vi "Command_verification_SA test.vi"(3 "time out":i32=40000, 4 "connection ID":refnum<k5>) -> (0 "Get_mea_condition":T1 {"RoiLateralSpan" format="%.2f"; "RoiLateralMin" format="%.2f"}, 1 "RLE data":string)   [LabVIEW 2016]
uses:
  TemperatureMeasure/Thermal_type.vi
panel:
  out "B-mode(Hout_Lout_Reg)":string[](array[string])
  in  "mea_condition_setting":T1 {"RoiLateralMin" format="%.2f"; "RoiLateralSpan" format="%.2f"}
  in  "error out":errorcluster
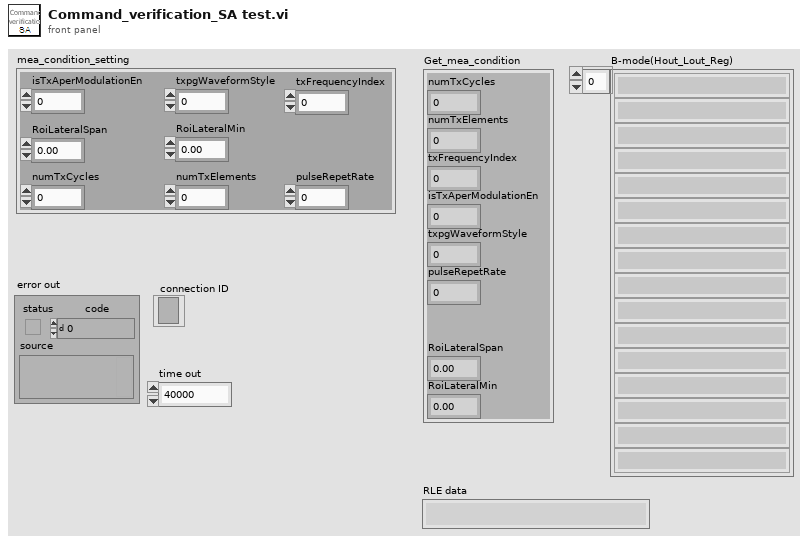
[diagram p1: front panel]
types:
  T1 = cluster{"numTxCycles":dbl, "numTxElements":i16, "txFrequencyIndex":i32, "isTxAperModulationEn":i16, "txpgWaveformStyle":i16, "pulseRepetRate":dbl, "RoiLateralSpan":dbl, "RoiLateralMin":dbl}
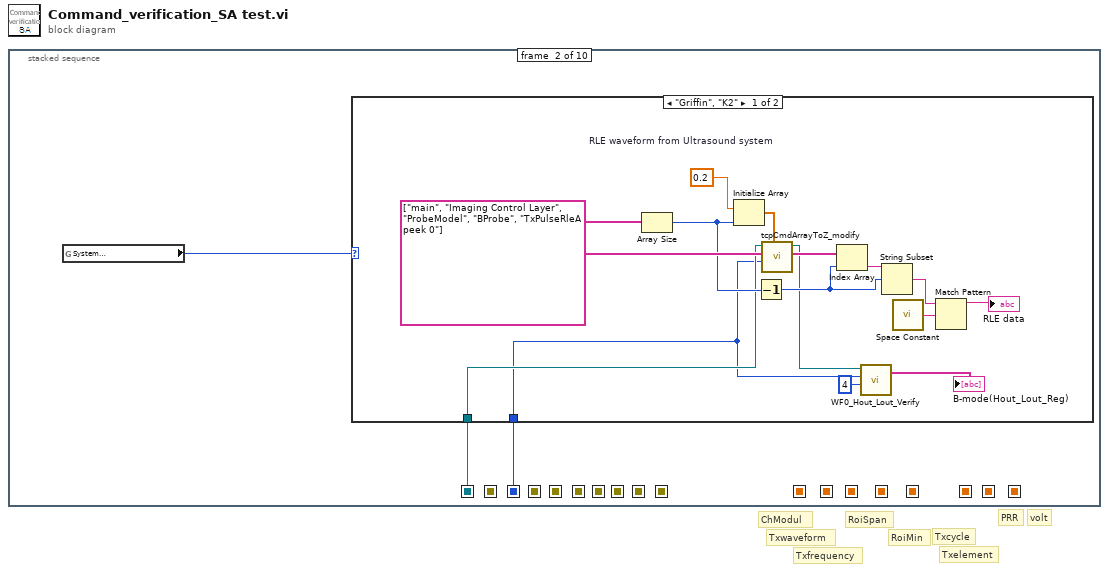
[diagram p0: block diagram]
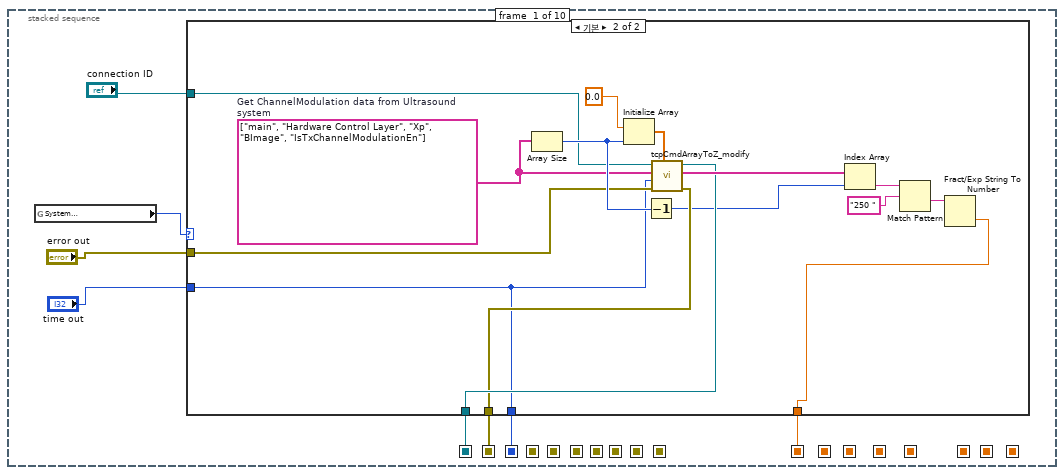
[diagram p2: hidden frame]
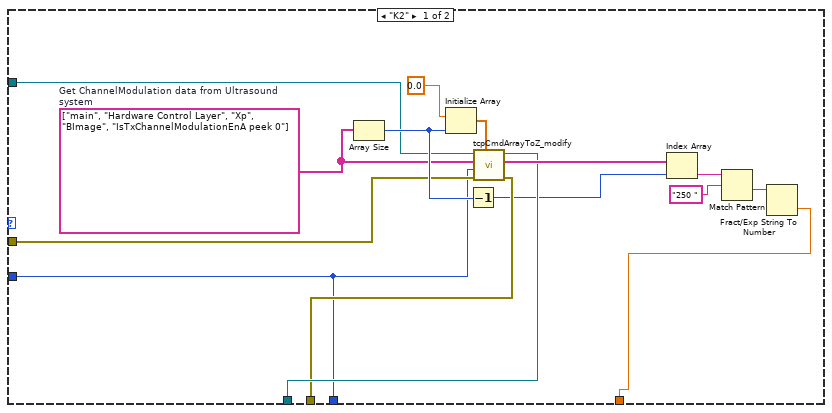
[diagram p3: hidden frame]
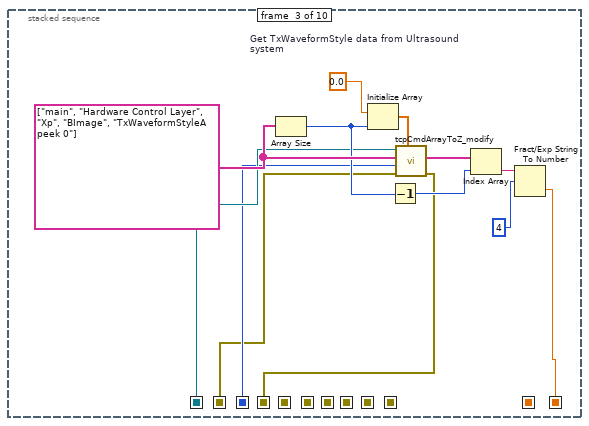
[diagram p5: hidden frame]
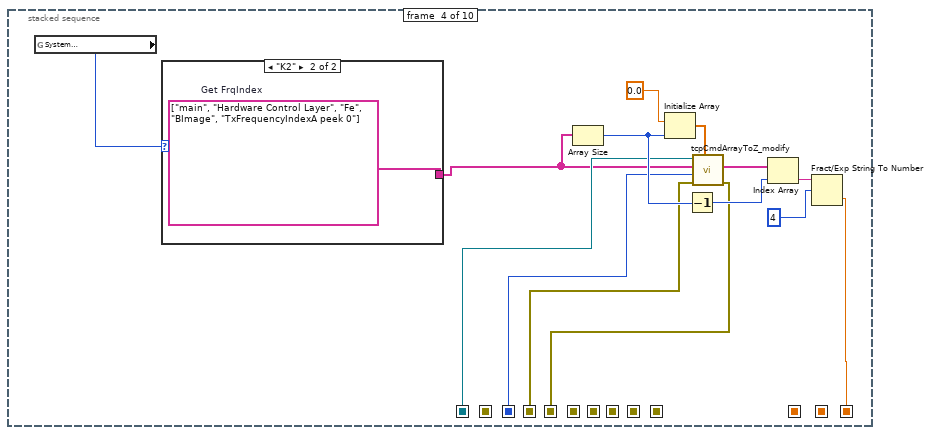
[diagram p6: hidden frame]
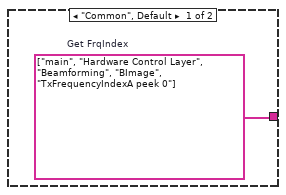
[diagram p7: hidden frame]
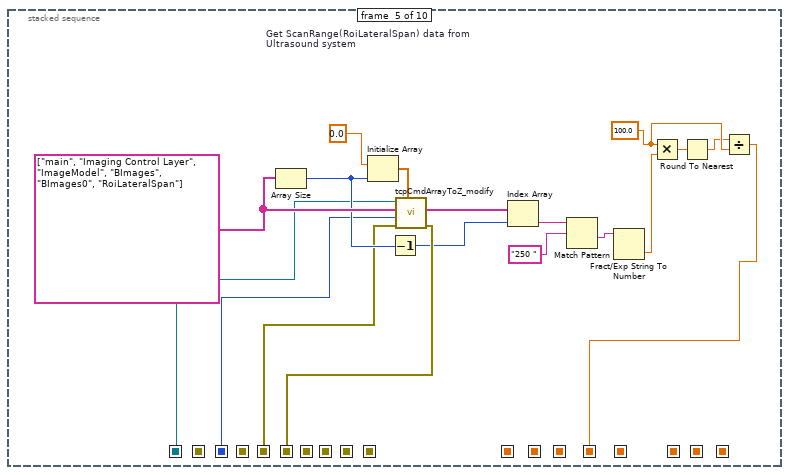
[diagram p8: hidden frame]
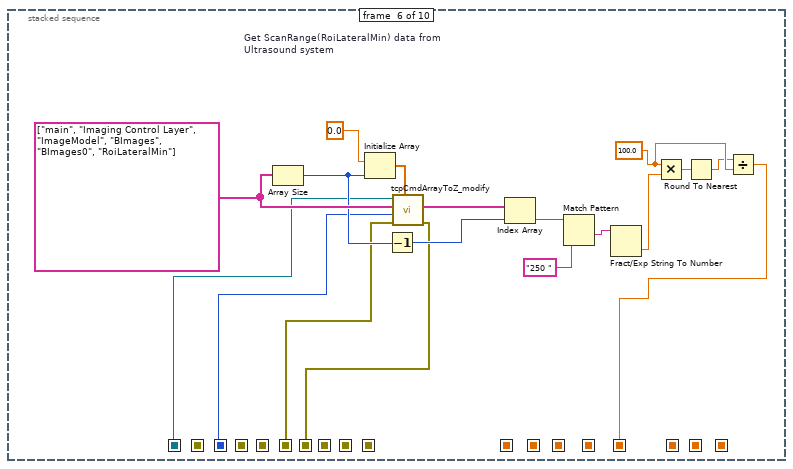
[diagram p9: hidden frame]
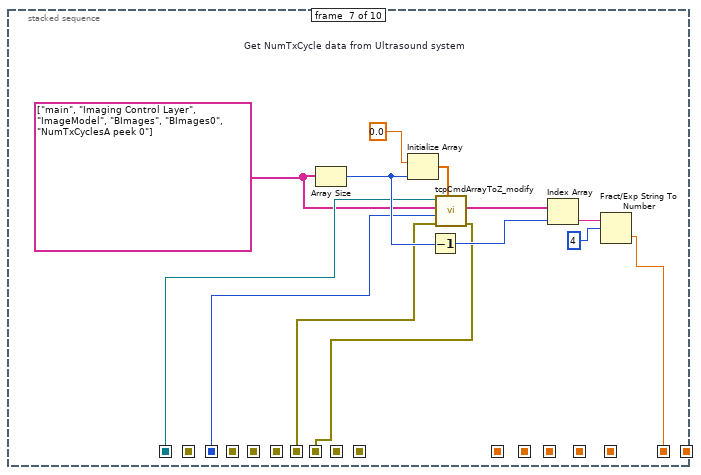
[diagram p10: hidden frame]
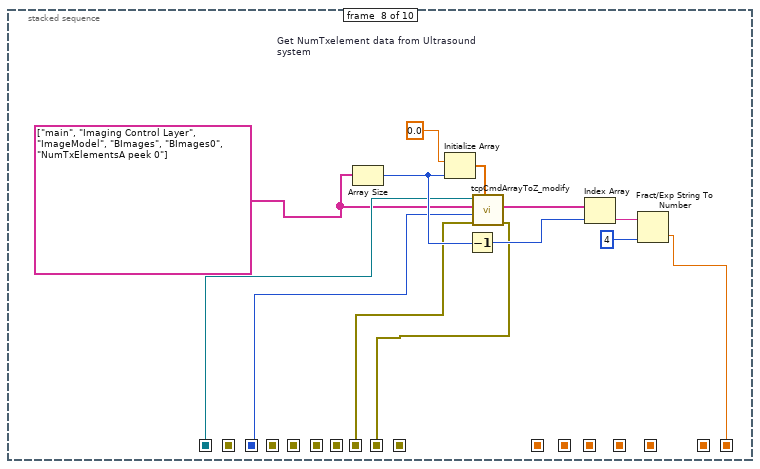
[diagram p11: hidden frame]
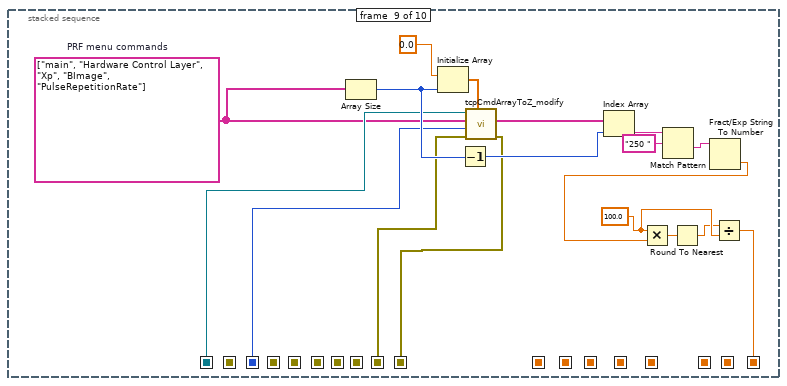
[diagram p12: hidden frame]
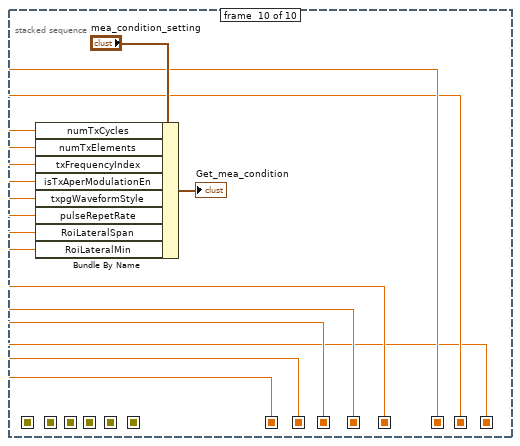
[diagram p13: hidden frame]
diagram:
  # "volt"
  # "PRR"
  # "Txelement"
  # "Txcycle"
  # "RoiMin"
  # "RoiSpan"
  # "Txfrequency"
  # "Txwaveform"
  # "ChModul"
  n1 = stacked-sequence {
    seq-local: [w8 _ _ _ _ _ _ _ _ _] -> [_ _ _ _ _ _ _ _ _ w174]
    seq-local: [w7 _ _ _ _ _ _ _ _ _] -> [_ w41 w64 w76 w99 w114 w128 w141 w162 _]
    seq-local: [w6 _ _ _ _ _ _ _ _ _] -> [_ _ w62 _ _ _ _ _ _ _]
    seq-local: [w5 _ _ _ _ _ _ _ _ _] -> [_ w40 w63 w75 w98 w113 w127 w140 w161 _]
    seq-local: [_ _ w59 _ _ _ _ _ _ _] -> [_ _ _ _ _ _ _ _ _ w173]
    seq-local: [_ _ w58 _ _ _ _ _ _ _] -> [_ _ _ w74 _ _ _ _ _ _]
    seq-local: [_ _ _ w77 _ _ _ _ _ _] -> [_ _ _ _ _ _ _ _ _ w172]
    seq-local: [_ _ _ w73 _ _ _ _ _ _] -> [_ _ _ _ w97 _ _ _ _ _]
    seq-local: [_ _ _ _ w96 _ _ _ _ _] -> [_ _ _ _ _ w112 _ _ _ _]
    seq-local: [_ _ _ _ w86 _ _ _ _ _] -> [_ _ _ _ _ _ _ _ _ w171]
    seq-local: [_ _ _ _ _ w111 _ _ _ _] -> [_ _ _ _ _ _ w123 _ _ _]
    seq-local: [_ _ _ _ _ w104 _ _ _ _] -> [_ _ _ _ _ _ _ _ _ w170]
    seq-local: [_ _ _ _ _ _ w122 _ _ _] -> [_ _ _ _ _ _ _ w136 _ _]
    seq-local: [_ _ _ _ _ _ _ w135 _ _] -> [_ _ _ _ _ _ _ _ w149 _]
    seq-local: [_ _ _ _ _ _ w126 _ _ _] -> [_ _ _ _ _ _ _ _ _ w169]
    seq-local: [_ _ _ _ _ _ _ _ w148 _] -> [_ _ _ _ _ _ _ _ _ _]
    seq-local: [_ _ _ _ _ _ _ w139 _ _] -> [_ _ _ _ _ _ _ _ _ w168]
    seq-local: [_ _ _ _ _ _ _ _ w150 _] -> [_ _ _ _ _ _ _ _ _ w167]
    frame #0 {
      n2 = global read "Thermal_type.vi" "System \nSelection"() -> (w4:enum32{"Common", "Frosk", "Griffin", "K2"})
      n3 = case shown="기본" w4 {
        tunnel: [w18 w33] -> w8
        tunnel: [w17 w32] -> w7
        tunnel: [w16 w31] -> w6
        tunnel: [w9 w24] -> w5
        tunnel: "connection ID" -> [w11 w26]
        tunnel: "error out" -> [w10 w25]
        tunnel: "time out" -> [w9 w24]
        frame "K2" {
          w15 = string[] ["main", "Hardware Control Layer", "Xp", "BImage", "IsTxChannelModulationEnA peek 0"]  # Get ChannelModulation data from Ultrasound system
          n4 = Array Size(array=w15) -> (size(s)=w20:i32)
          n5 = Initialize Array(0.0 ("원소"), w20) -> (w22:dbl[])
          n6 = Decrement(x=w20) -> (x-1=w14:i32)
          n7 = call "tcpCmdArrayToZ_modify.vi"("Delay (sec)"=w22, "error in (no error)"=w10, "Timeout (ms)"=w9, "Command array"=w15, "connection ID in"=w11) -> ("error out"=w16:errorcluster, "Receive array"=w21:string[], "connection ID out"=w17:refnum<k5>)  [unwired: 2 in, 2 out]
          n8 = Index Array(array=w21, index=w14) -> (element=w19:string)
          n9 = Match Pattern(string=w19, regular expression="250 " ("정규식")) -> (after substring=w13:string)  [unwired: 1 in, 3 out]
          n10 = Fract/Exp String To Number(string=w13) -> (number=w18:dbl)  [unwired: 3 in, 1 out]
        }
        frame Default {
          w30 = string[] ["main", "Hardware Control Layer", "Xp", "BImage", "IsTxChannelModulationEn"]  # Get ChannelModulation data from Ultrasound system
          n11 = Array Size(array=w30) -> (size(s)=w35:i32)
          n12 = Initialize Array(0.0 ("원소"), w35) -> (w37:dbl[])
          n13 = Decrement(x=w35) -> (x-1=w29:i32)
          n14 = call "tcpCmdArrayToZ_modify.vi"("Delay (sec)"=w37, "error in (no error)"=w25, "Timeout (ms)"=w24, "Command array"=w30, "connection ID in"=w26) -> ("error out"=w31:errorcluster, "Receive array"=w36:string[], "connection ID out"=w32:refnum<k5>)  [unwired: 2 in, 2 out]
          n15 = Index Array(array=w36, index=w29) -> (element=w34:string)
          n16 = Match Pattern(string=w34, regular expression="250 " ("정규식")) -> (after substring=w28:string)  [unwired: 1 in, 3 out]
          n17 = Fract/Exp String To Number(string=w28) -> (number=w33:dbl)  [unwired: 3 in, 1 out]
        }
      }
    }
    frame #1 {
      n18 = global read "Thermal_type.vi" "System \nSelection"() -> (w39:enum32{"Common", "Frosk", "Griffin", "K2"})
      n19 = case shown="\"Griffin\", \"K2\"" w39 {
        tunnel: w41 -> [w46 _]
        tunnel: w40 -> [w44 _]
        frame "Griffin", "K2" {
          w56 = string[] ["main", "Imaging Control Layer", "ProbeModel", "BProbe", "TxPulseRleA peek 0"]  # RLE waveform from Ultrasound system
          n20 = Array Size(array=w56) -> (size(s)=w52:i32)
          n21 = Initialize Array(0.2 ("원소"), w52) -> (w54:dbl[])
          n22 = Decrement(x=w52) -> (x-1=w50:i32)
          n23 = call "tcpCmdArrayToZ_modify.vi"("Delay (sec)"=w54, "Timeout (ms)"=w44, "Command array"=w56, "connection ID in"=w46) -> ("Receive array"=w53:string[], "connection ID out"=w45:refnum<k5>)  [unwired: 3 in, 3 out]
          n24 = Index Array(array=w53, index=w50) -> (element=w51:string)
          n25 = call "WF0_Hout_Lout_Verify.vi"("connection ID"=w45, "time out"=w44, "Num_Verify"=4) -> ("B-mode(Hout_Lout_Reg)"=→"B-mode(Hout_Lout_Reg)":string[])  [unwired: 1 in, 5 out]
          n26 = String Subset(string=w51, offset (0)=w50) -> (substring=w49:string)  [unwired: 1 in]
          n27 = call <vilib>:"Space Constant.vi"() -> ("String"=w48:string)
          n28 = Match Pattern(string=w49, regular expression=w48) -> (before substring=→"RLE data":string)  [unwired: 1 in, 3 out]
        }
        frame Default {
        }
      }
    }
    frame #2 {
      w69 = string[] ["main", "Hardware Control Layer", "Xp", "BImage", "TxWaveformStyleA peek 0"]  # Get TxWaveformStyle data from Ultrasound system
      n29 = Array Size(array=w69) -> (size(s)=w65:i32)
      n30 = Initialize Array(0.0 ("원소"), w65) -> (w67:dbl[])
      n31 = Decrement(x=w65) -> (x-1=w60:i32)
      n32 = call "tcpCmdArrayToZ_modify.vi"("Delay (sec)"=w67, "error in (no error)"=w62, "Timeout (ms)"=w63, "Command array"=w69, "connection ID in"=w64) -> ("error out"=w58:errorcluster, "Receive array"=w66:string[])  [unwired: 2 in, 3 out]
      n33 = Index Array(array=w66, index=w60) -> (element=w61:string)
      n34 = Fract/Exp String To Number(string=w61, offset=4 ("오프셋")) -> (number=w59:dbl)  [unwired: 2 in, 1 out]
    }
    frame #3 {
      n35 = global read "Thermal_type.vi" "System \nSelection"() -> (w71:enum32{"Common", "Frosk", "Griffin", "K2"})
      n36 = case shown="\"K2\"" w71 {
        tunnel: [w84 w85] -> w70
        frame "Common", Default {
          w84 = string[] ["main", "Hardware Control Layer", "Beamforming", "BImage", "TxFrequencyIndexA peek 0"]  # Get FrqIndex
        }
        frame "K2" {
          w85 = string[] ["main", "Hardware Control Layer", "Fe", "BImage", "TxFrequencyIndexA peek 0"]  # Get FrqIndex
        }
      }
      n37 = Array Size(array=w70) -> (size(s)=w80:i32)
      n38 = Initialize Array(0.0 ("원소"), w80) -> (w82:dbl[])
      n39 = Decrement(x=w80) -> (x-1=w78:i32)
      n40 = call "tcpCmdArrayToZ_modify.vi"("Delay (sec)"=w82, "error in (no error)"=w74, "Timeout (ms)"=w75, "Command array"=w70, "connection ID in"=w76) -> ("error out"=w73:errorcluster, "Receive array"=w81:string[])  [unwired: 2 in, 3 out]
      n41 = Index Array(array=w81, index=w78) -> (element=w79:string)
      n42 = Fract/Exp String To Number(string=w79, offset=4 ("오프셋")) -> (number=w77:dbl)  [unwired: 2 in, 1 out]
    }
    frame #4 {
      w89 = 100.0
      w103 = string[] ["main", "Imaging Control Layer", "ImageModel", "BImages", "BImages0", "RoiLateralSpan"]  # Get ScanRange(RoiLateralSpan) data from Ultrasound system
      n43 = Array Size(array=w103) -> (size(s)=w100:i32)
      n44 = Initialize Array(0.0 ("원소"), w100) -> (w101:dbl[])
      n45 = Decrement(x=w100) -> (x-1=w93:i32)
      n46 = call "tcpCmdArrayToZ_modify.vi"("Delay (sec)"=w101, "error in (no error)"=w97, "Timeout (ms)"=w98, "Command array"=w103, "connection ID in"=w99) -> ("error out"=w96:errorcluster, "Receive array"=w94:string[])  [unwired: 2 in, 3 out]
      n47 = Index Array(array=w94, index=w93) -> (element=w95:string)
      n48 = Match Pattern(string=w95, regular expression="250 " ("정규식")) -> (after substring=w92:string)  [unwired: 1 in, 3 out]
      n49 = Fract/Exp String To Number(string=w92) -> (number=w87:dbl)  [unwired: 3 in, 1 out]
      n50 = Multiply(x=w89, y=w87) -> (x*y=w90:dbl)
      n51 = Round To Nearest(number=w90) -> (nearest integer value=w88:dbl)
      n52 = Divide(x=w88, y=w89) -> (x/y=w86:dbl)
    }
    frame #5 {
      w107 = 100.0
      w121 = string[] ["main", "Imaging Control Layer", "ImageModel", "BImages", "BImages0", "RoiLateralMin"]  # Get ScanRange(RoiLateralMin) data from Ultrasound system
      n53 = Array Size(array=w121) -> (size(s)=w118:i32)
      n54 = Initialize Array(0.0 ("원소"), w118) -> (w119:dbl[])
      n55 = Decrement(x=w118) -> (x-1=w115:i32)
      n56 = call "tcpCmdArrayToZ_modify.vi"("Delay (sec)"=w119, "error in (no error)"=w112, "Timeout (ms)"=w113, "Command array"=w121, "connection ID in"=w114) -> ("error out"=w111:errorcluster, "Receive array"=w116:string[])  [unwired: 2 in, 3 out]
      n57 = Index Array(array=w116, index=w115) -> (element=w117:string)
      n58 = Match Pattern(string=w117, regular expression="250 " ("정규식")) -> (after substring=w109:string)  [unwired: 1 in, 3 out]
      n59 = Fract/Exp String To Number(string=w109) -> (number=w105:dbl)  [unwired: 3 in, 1 out]
      n60 = Multiply(x=w107, y=w105) -> (x*y=w108:dbl)
      n61 = Round To Nearest(number=w108) -> (nearest integer value=w106:dbl)
      n62 = Divide(x=w106, y=w107) -> (x/y=w104:dbl)
    }
    frame #6 {
      w125 = string[] ["main", "Imaging Control Layer", "ImageModel", "BImages", "BImages0", "NumTxCyclesA peek 0"]  # Get NumTxCycle data from Ultrasound system
      n63 = Array Size(array=w125) -> (size(s)=w132:i32)
      n64 = Initialize Array(0.0 ("원소"), w132) -> (w133:dbl[])
      n65 = Decrement(x=w132) -> (x-1=w129:i32)
      n66 = call "tcpCmdArrayToZ_modify.vi"("Delay (sec)"=w133, "error in (no error)"=w123, "Timeout (ms)"=w127, "Command array"=w125, "connection ID in"=w128) -> ("error out"=w122:errorcluster, "Receive array"=w131:string[])  [unwired: 2 in, 3 out]
      n67 = Index Array(array=w131, index=w129) -> (element=w130:string)
      n68 = Fract/Exp String To Number(string=w130, offset=4 ("오프셋")) -> (number=w126:dbl)  [unwired: 2 in, 1 out]
    }
    frame #7 {
      w138 = string[] ["main", "Imaging Control Layer", "ImageModel", "BImages", "BImages0", "NumTxElementsA peek 0"]  # Get NumTxelement data from Ultrasound system
      n69 = Array Size(array=w138) -> (size(s)=w145:i32)
      n70 = Initialize Array(0.0 ("원소"), w145) -> (w146:dbl[])
      n71 = Decrement(x=w145) -> (x-1=w142:i32)
      n72 = call "tcpCmdArrayToZ_modify.vi"("Delay (sec)"=w146, "error in (no error)"=w136, "Timeout (ms)"=w140, "Command array"=w138, "connection ID in"=w141) -> ("error out"=w135:errorcluster, "Receive array"=w144:string[])  [unwired: 2 in, 3 out]
      n73 = Index Array(array=w144, index=w142) -> (element=w143:string)
      n74 = Fract/Exp String To Number(string=w143, offset=4 ("오프셋")) -> (number=w139:dbl)  [unwired: 2 in, 1 out]
    }
    frame #8 {
      w153 = 100.0
      w160 = string[] ["main", "Hardware Control Layer", "Xp", "BImage", "PulseRepetitionRate"]  # PRF menu commands
      n75 = Array Size(array=w160) -> (size(s)=w163:i32)
      n76 = Initialize Array(0.0 ("원소"), w163) -> (w164:dbl[])
      n77 = Decrement(x=w163) -> (x-1=w158:i32)
      n78 = call "tcpCmdArrayToZ_modify.vi"("Delay (sec)"=w164, "error in (no error)"=w149, "Timeout (ms)"=w161, "Command array"=w160, "connection ID in"=w162) -> ("error out"=w148:errorcluster, "Receive array"=w159:string[])  [unwired: 2 in, 3 out]
      n79 = Index Array(array=w159, index=w158) -> (element=w157:string)
      n80 = Match Pattern(string=w157, regular expression="250 " ("정규식")) -> (after substring=w155:string)  [unwired: 1 in, 3 out]
      n81 = Fract/Exp String To Number(string=w155) -> (number=w151:dbl)  [unwired: 3 in, 1 out]
      n82 = Multiply(x=w153, y=w151) -> (x*y=w154:dbl)
      n83 = Round To Nearest(number=w154) -> (nearest integer value=w152:dbl)
      n84 = Divide(x=w152, y=w153) -> (x/y=w150:dbl)
    }
    frame #9 {
      n85 = Bundle By Name(cluster="mea_condition_setting", "numTxCycles"=w169, "numTxElements"=w168, "txFrequencyIndex"=w172, "isTxAperModulationEn"=w174, "txpgWaveformStyle"=w173, "pulseRepetRate"=w167, "RoiLateralSpan"=w171, "RoiLateralMin"=w170) -> (→"Get_mea_condition":T1)
    }
  }
